vi "CMN_buildImageName.vi"(6 "Database RefNum out":T1, 7 "Path":path, 8 "imageNumber":i32, 9 "root name":string) -> (0 "Path out":path, 1 "image":string, 2 "output root":string, 3 "image name":string, 4 "number":i32)   [LabVIEW 2016]
uses:
  DBSHAND/private/vis/DatabaseHand_RefNum.ctl
  DBSHAND/private/vis/DatabaseHand_Element_Get(I32).vi
  DBSHAND/private/vis/DatabaseHand_Element_Get(string).vi
  DBSHAND/private/vis/DatabaseHand_Element_Get(bool).vi
  DBSHAND/private/vis/DatabaseHand_Element_Set(I32).vi
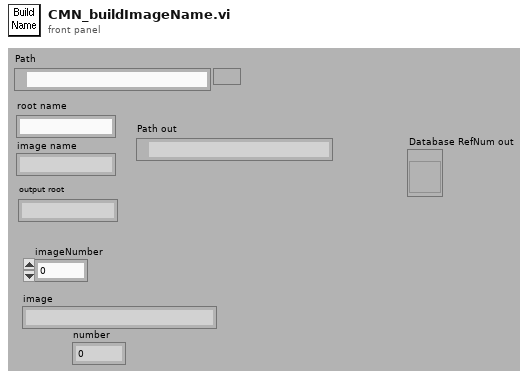
[diagram p1: front panel]
types:
  T1 = typedef "DatabaseHand_RefNum.ctl" = refnum<vi>
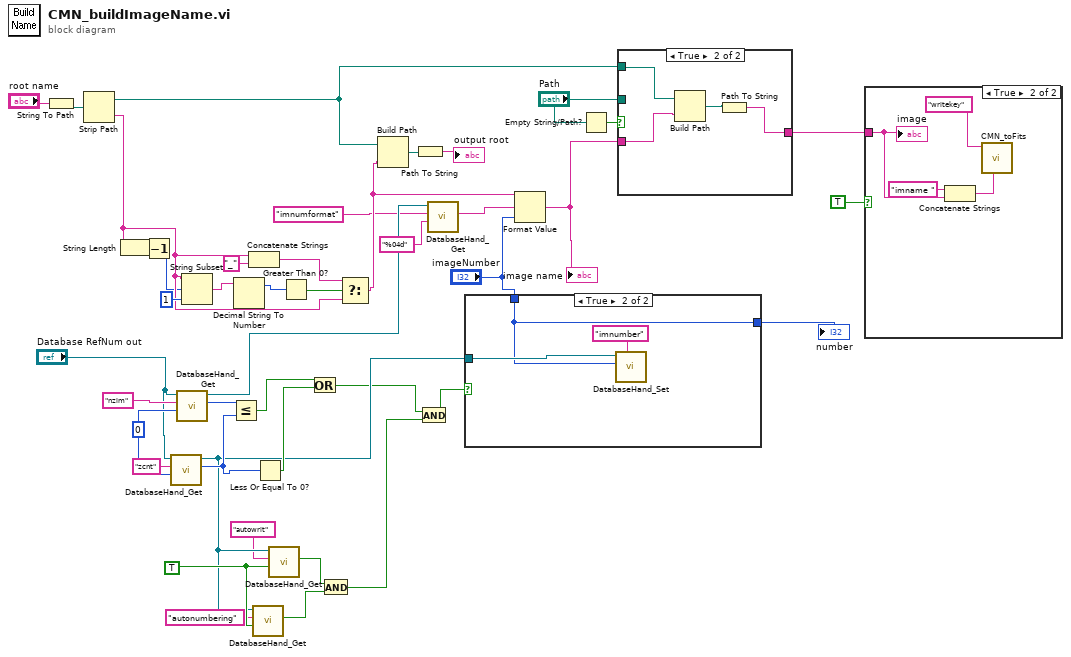
[diagram p0: block diagram]
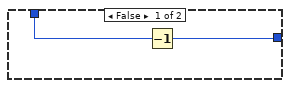
[diagram p3: hidden frame]
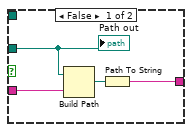
[diagram p4: hidden frame]
diagram:
  w9 = TRUE
  w19 = 0
  n1 = String To Path(string="root name") -> (path=w40:path)
  n2 = Strip Path(path=w40) -> (stripped path=w38:path, name=w28:string)
  n3 = String Length(string=w28) -> (length=w35:i32)
  n4 = Decrement(x=w35) -> (x-1=w26:i32)
  n5 = call-poly "DatabaseHand_Get.vi"("default value"=w19, "name"="zcnt", "Database RefNum in"="Database RefNum out") -> ("value"=w18:i32, "Database RefNum out"=w6:T1)  [unwired: 2 in, 5 out]
  n6 = call-poly "DatabaseHand_Get.vi"("default value"=w19, "name"="nzim", "Database RefNum in"="Database RefNum out") -> ("value"=w23:i32, "Database RefNum out"=w14:T1)  [unwired: 2 in, 5 out]
  n7 = String Subset(string=w28, offset (0)=w26, length (rest)=1 ("length (rest)")) -> (substring=w33:string)
  n8 = Less Or Equal?(x=w23, y=w18) -> (x <= y?=w22:bool)
  n9 = Decimal String To Number(string=w33) -> (offset past number=w32:i32)  [unwired: 3 out]
  n10 = Concatenate Strings(w28, "_" ("string")) -> (w29:string)
  n11 = call-poly "DatabaseHand_Get.vi"("default value"=w9, "name"="autonumbering", "Database RefNum in"=w6) -> ("value"=w7:bool)  [unwired: 2 in, 6 out]
  n12 = Less Or Equal To 0?(x=w18) -> (x <= 0?=w21:bool)
  n13 = call-poly "DatabaseHand_Get.vi"("default value"=w9, "name"="autowrit", "Database RefNum in"=w6) -> ("value"=w10:bool)  [unwired: 2 in, 6 out]
  n14 = Greater Than 0?(x=w32) -> (x > 0?=w31:bool)
  n15 = Or(x=w22, y=w21) -> (x .or. y?=w3:bool)
  n16 = And(x=w10, y=w7) -> (x .and. y?=w4:bool)
  n17 = Select(t=w29, s=w31, f=w28) -> (s? t:f=w27:string)
  n18 = Build Path(base path=w38, name or relative path=w27) -> (appended path=w37:path)
  n19 = Path To String(path=w37) -> (string=→"output root":string)
  n20 = And(x=w3, y=w4) -> (x .and. y?=w2:bool)
  n21 = call-poly "DatabaseHand_Get.vi"("default value"="%04d" ("format string"), "name"="imnumformat", "Database RefNum in"=w14) -> ("value"=w11:string)  [unwired: 2 in, 6 out]
  n22 = case shown="True" w2 {
    tunnel: w6 -> [_ w47]
    tunnel: "imageNumber" -> [w45 w46]
    tunnel: [w44 w46] -> w15
    frame False {
      n23 = Decrement(x=w45) -> (x-1=w44:i32)
    }
    frame True {
      n24 = call-poly "DatabaseHand_Set.vi"("name"="imnumber", "value"=w46, "Database RefNum in"=w47) -> ()  [unwired: 5 in, 4 out]
    }
  }
  "number" <- w15
  n25 = Format Value(string ("")=w27, format string=w11, value (0)="imageNumber") -> (output string=w42:string)
  "image name" <- w42
  n26 = Empty String/Path?(string/path="Path") -> (empty?=w43:bool)
  n27 = case shown="True" w43 {
    tunnel: w42 -> [w52 w55]
    tunnel: "Path" -> [w50 _]
    tunnel: [w49 w53] -> w25
    tunnel: w38 -> [_ w56]
    frame False {
      n28 = Build Path(base path=w50, name or relative path=w52) -> (appended path=w51:path)
      n29 = Path To String(path=w51) -> (string=w49:string)
      "Path out" <- w50
    }
    frame True {
      n30 = Build Path(base path=w56, name or relative path=w55) -> (appended path=w54:path)
      n31 = Path To String(path=w54) -> (string=w53:string)
    }
  }
  n32 = case shown="True" TRUE {
    tunnel: w25 -> [_ w58]
    frame False {
    }
    frame True {
      n33 = Concatenate Strings("imname " ("string"), w58) -> (w57:string)
      n34 = call "CMN_toFits.vi"("key"=w57, "command"="writekey") -> ()  [unwired: 6 in, 4 out]
      "image" <- w58
    }
  }
